vi "IMSetup.vi"(0 "VISA IN":refnum<visa-resource-name>, 1 "F1":dbl, 2 "F2":dbl, 5 "error in":errorcluster, 6 "Autoscale?":bool=TRUE, 7 "Channel":i32=1, 8 "Filename":string="INTERMOD", 9 "Window":i32=1, 11 "Trace":i32=1) -> (14 "VISA Out":refnum<visa-resource-name>, 19 "error out":errorcluster)   [LabVIEW 2018]
uses:
  PNA-X.lvlib
panel:
  in  "AVG Factor":i32=20
  in  "Average?":bool=TRUE
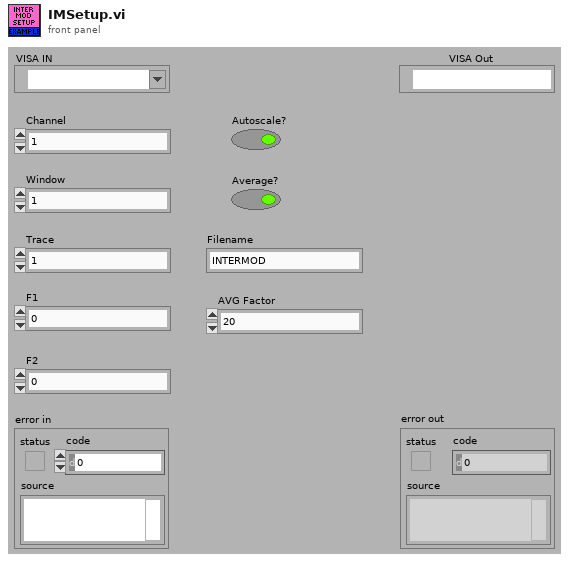
[diagram p1: front panel]
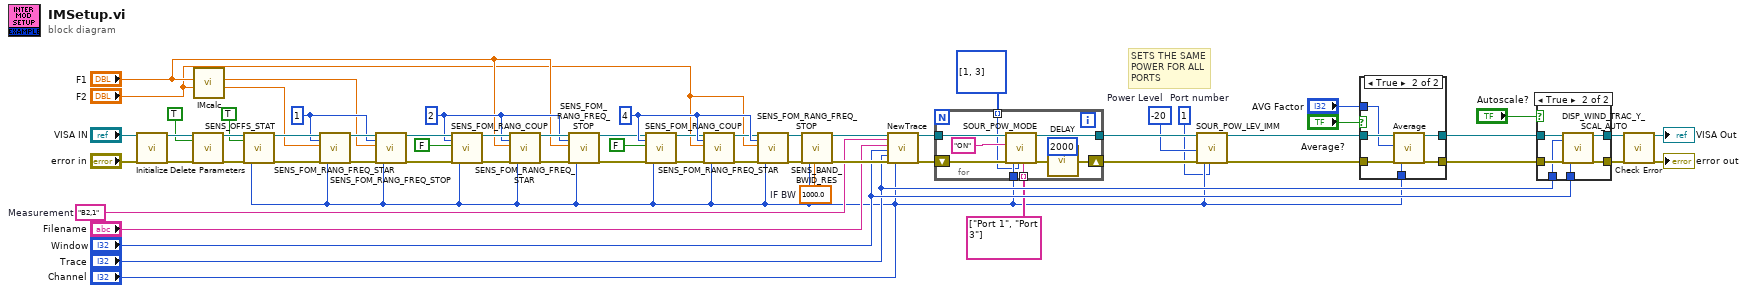
[diagram p0: block diagram]
diagram:
  w17 = -20  # Power Level
  w1 = 1  # Port number
  w32 = 4 ("Range number")
  w33 = 2 ("Range number")
  w41 = 1 ("Range number")
  w49 = "B2,1"  # Measurement
  w53 = 1000.0  # IF BW
  # "SETS THE SAME POWER FOR ALL PORTS"
  n1 = call "Initialize.vi"("VISA IN"="VISA IN", "error in"="error in") -> ("VISA Out"=w62:refnum<visa-resource-name>, "error out"=w60:errorcluster)  [unwired: 15 in, 1 out]
  n2 = call "Delete Parameters .vi"("VISA IN"=w62, "Delete All?"=TRUE, "error in"=w60) -> ("VISA Out"=w47:refnum<visa-resource-name>, "error out"=w46:errorcluster)  [unwired: 15 in]
  n3 = call "IMcalc.vi"("F2"="F2", "F1"="F1") -> ("LIM"=w5:dbl, "UIM"=w4:dbl)  [unwired: 4 in]
  n4 = call "SENS_OFFS_STAT.vi"("VISA IN"=w47, "Frq. Offset ON/OFF"=TRUE, "error in"=w46, "Channel"="Channel") -> ("VISA Out"=w43:refnum<visa-resource-name>, "error out"=w45:errorcluster)  [unwired: 14 in]
  n5 = call "SENS_FOM_RANG_FREQ_STAR.vi"("VISA IN"=w43, "Range number"=w41, "Frq. Start"=w5, "error in"=w45, "Channel"="Channel") -> ("VISA Out"=w42:refnum<visa-resource-name>, "error out"=w44:errorcluster)  [unwired: 13 in]
  n6 = call "SENS_FOM_RANG_FREQ_STOP.vi"("VISA IN"=w42, "Range number"=w41, "Frq. Stop"=w4, "error in"=w44, "Channel"="Channel") -> ("VISA Out"=w40:refnum<visa-resource-name>, "error out"=w39:errorcluster)  [unwired: 13 in]
  n7 = call "SENS_FOM_RANG_COUP.vi"("VISA IN"=w40, "Range number"=w33, "Couple Range to Primary Range ON/OFF"=FALSE, "error in"=w39, "Channel"="Channel") -> ("VISA Out"=w37:refnum<visa-resource-name>, "error out"=w36:errorcluster)  [unwired: 13 in]
  n8 = call "SENS_FOM_RANG_FREQ_STAR.vi"("VISA IN"=w37, "Range number"=w33, "Frq. Start"="F1", "error in"=w36, "Channel"="Channel") -> ("VISA Out"=w34:refnum<visa-resource-name>, "error out"=w35:errorcluster)  [unwired: 13 in]
  n9 = call "SENS_FOM_RANG_FREQ_STOP.vi"("VISA IN"=w34, "Range number"=w33, "Frq. Stop"="F1", "error in"=w35, "Channel"="Channel") -> ("VISA Out"=w26:refnum<visa-resource-name>, "error out"=w25:errorcluster)  [unwired: 13 in]
  n10 = call "SENS_FOM_RANG_COUP.vi"("VISA IN"=w26, "Range number"=w32, "Couple Range to Primary Range ON/OFF"=FALSE, "error in"=w25, "Channel"="Channel") -> ("VISA Out"=w28:refnum<visa-resource-name>, "error out"=w29:errorcluster)  [unwired: 13 in]
  n11 = call "SENS_FOM_RANG_FREQ_STAR.vi"("VISA IN"=w28, "Range number"=w32, "Frq. Start"="F2", "error in"=w29, "Channel"="Channel") -> ("VISA Out"=w31:refnum<visa-resource-name>, "error out"=w30:errorcluster)  [unwired: 13 in]
  n12 = call "SENS_FOM_RANG_FREQ_STOP.vi"("VISA IN"=w31, "Range number"=w32, "Frq. Stop"="F2", "error in"=w30, "Channel"="Channel") -> ("VISA Out"=w24:refnum<visa-resource-name>, "error out"=w23:errorcluster)  [unwired: 13 in]
  n13 = call "SENS_BAND_BWID_RES.vi"("VISA IN"=w24, "error in"=w23, "Channel"="Channel", "Resolution"=w53) -> ("VISA Out"=w54:refnum<visa-resource-name>, "error out"=w55:errorcluster)  [unwired: 14 in]
  n14 = call "NewTrace.vi"("VISA IN"=w54, "Measurement"=w49, "FileName"="Filename", "Window"="Window", "Trace"="Trace", "error in (no error)"=w55, "Channel"="Channel") -> ("VISA Out"=w16:refnum<visa-resource-name>, "error out"=w15:errorcluster)  [unwired: 11 in]
  n15 = for {
    tunnel: w16 -> [w72]
    tunnel: [w68] -> w18
    tunnel: i32[] [1, 3] -> [w63] mode=indexing
    tunnel: string[] ["Port 1", "Port 3"] -> [w64] mode=indexing
    shift-right: [w67] -> w19
    shift-left: w15 -> [w71]
    tunnel: "Channel" -> [w65]
    n16 = call "SOUR_POW_MODE.vi"("VISA IN"=w72, "Source State"="ON", "error in"=w71, "Channel"=w65, "Port number"=w63, "Source"=w64) -> ("VISA Out"=w68:refnum<visa-resource-name>, "error out"=w69:errorcluster)  [unwired: 12 in]
    n17 = call "DELAY.vi"("milliseconds to wait"=u32 2000, "error in (no error)"=w69) -> ("error out"=w67:errorcluster)  [unwired: 13 in]
  }
  n18 = call "SOUR_POW_LEV_IMM.vi"("VISA IN"=w18, "Power Level"=w17, "error in"=w19, "Channel"="Channel", "Port number"=w1) -> ("VISA Out"=w7:refnum<visa-resource-name>, "error out"=w9:errorcluster)  [unwired: 13 in]
  n19 = case shown="True" "Average?" {
    tunnel: w7 -> [w74 w80]
    tunnel: w9 -> [w73 w79]
    tunnel: [w73 w78] -> w10
    tunnel: [w74 w77] -> w6
    tunnel: "Channel" -> [_ w76]
    tunnel: "AVG Factor" -> [_ w75]
    frame False {
    }
    frame True {
      n20 = call "Average.vi"("VISA IN"=w80, "AVG"=w75, "error in"=w79, "Channel"=w76) -> ("VISA Out"=w77:refnum<visa-resource-name>, "error out"=w78:errorcluster)  [unwired: 14 in]
    }
  }
  n21 = case shown="True" "Autoscale?" {
    tunnel: w10 -> [w82 w88]
    tunnel: w6 -> [w81 w87]
    tunnel: "Trace" -> [_ w86]
    tunnel: "Window" -> [_ w85]
    tunnel: [w81 w84] -> w13
    tunnel: [w82 w83] -> w14
    frame False {
    }
    frame True {
      n22 = call "DISP_WIND_TRAC_Y_SCAL_AUTO.vi"("VISA IN"=w87, "Trace"=w86, "error in"=w88, "Window"=w85) -> ("VISA Out"=w84:refnum<visa-resource-name>, "error out"=w83:errorcluster)  [unwired: 14 in]
    }
  }
  n23 = call "Check Error.vi"("VISA Resource Name"=w13, "error in (no error)"=w14) -> ("dup VISA session"=→"VISA Out":refnum<visa-resource-name>, "error out"=→"error out":errorcluster)  [unwired: 16 in]
